vi "Wind_Tunnel.vi"() -> ()   [LabVIEW 2025]
uses:
  <vilib>/express/express arith-compare/Formula/XNode/ExpressFormulaBlockNode.xnode
panel:
  out "mph":dbl
  out "10":dbl(graph)
  out "Waveform Chart 2":dbl(graph)
  out "5":dbl(graph)
  out "m/s":dbl
  out "Numeric":dbl
  out "ma 10":dbl
  out "?":dbl
  out "PSIG 10":dbl(knob) scale=-2.0..5.0
  out "ma 9":dbl
  out "?":dbl
  out "PSIG 9":dbl(knob) scale=-2.0..5.0
  out "ma 8":dbl
  out "?":dbl
  out "PSIG 8":dbl(knob) scale=-2.0..5.0
  out "ma 7":dbl
  out "?":dbl
  out "PSIG 7":dbl(knob) scale=-2.0..5.0
  out "ma 6":dbl
  out "?":dbl
  out "PSIG 6":dbl(knob) scale=-2.0..5.0
  out "ma 5":dbl
  out "?":dbl
  out "PSIG 5":dbl(knob) scale=-2.0..5.0
  out "ma 4":dbl
  out "?":dbl
  out "PSIG 4":dbl(knob) scale=-2.0..5.0
  out "ma 3":dbl
  out "?":dbl
  out "PSIG 3":dbl(knob) scale=-2.0..5.0
  out "ma 2":dbl
  out "?":dbl
  out "PSIG 2":dbl(knob) scale=-2.0..5.0
  out "ma":dbl
  out "?":dbl
  out "PSIG":dbl(knob) scale=-2.0..5.0
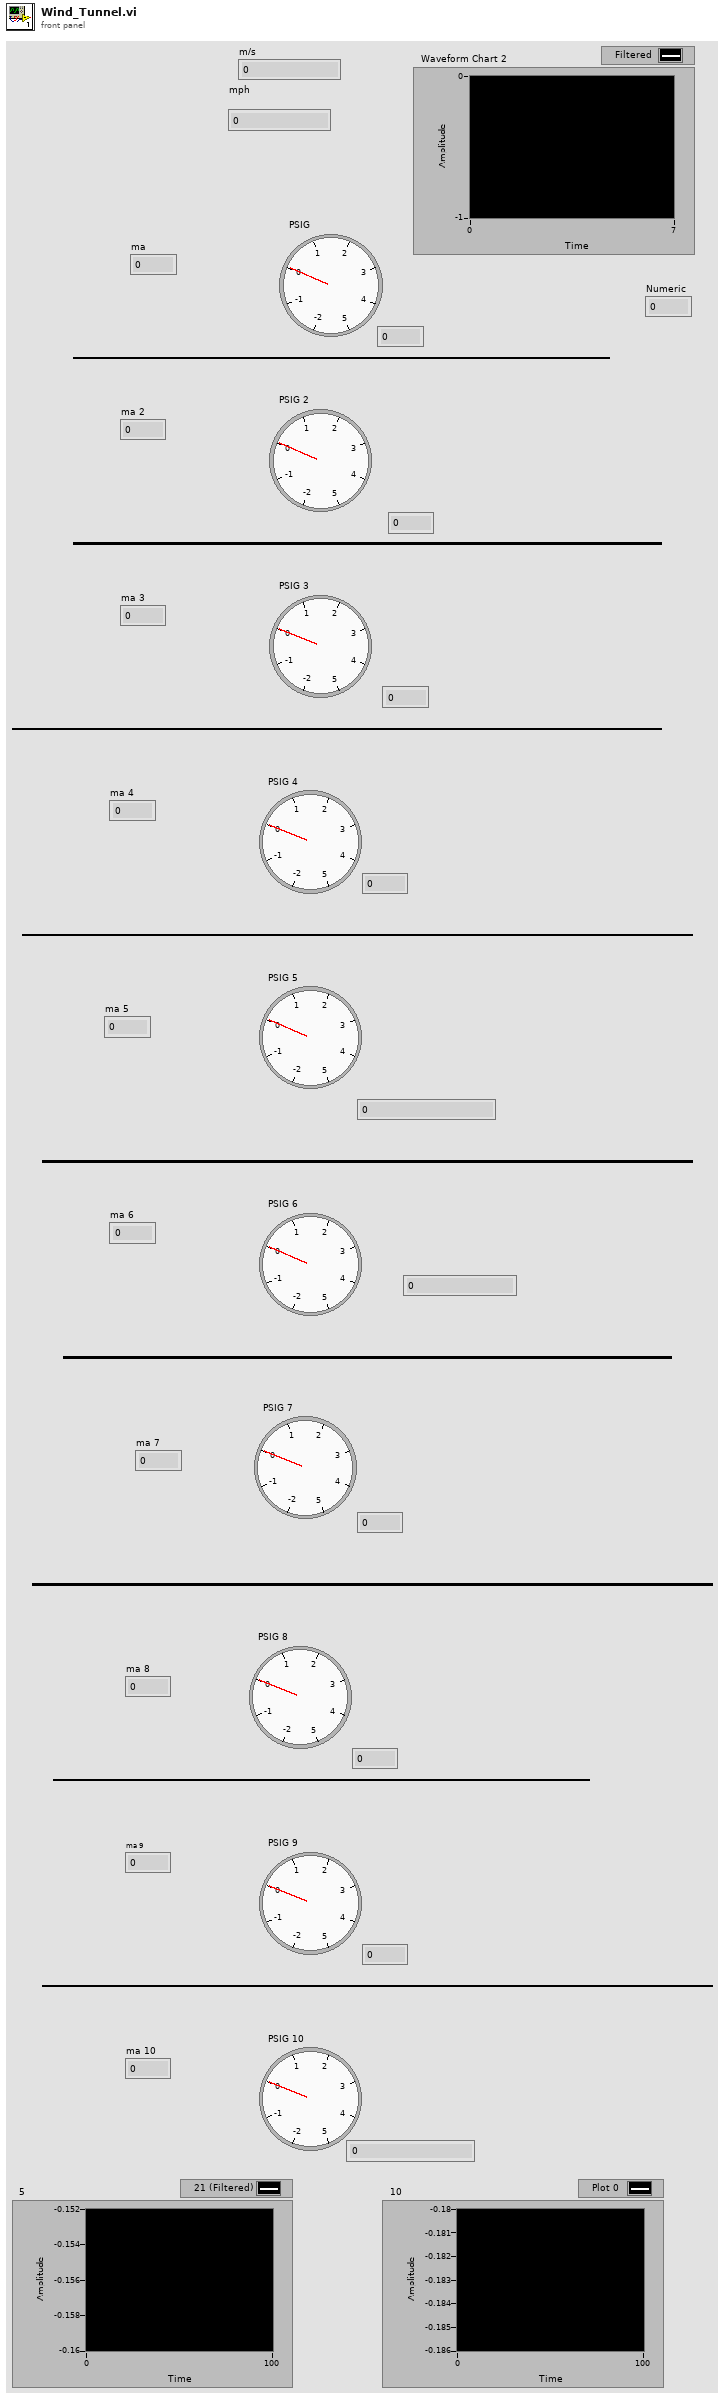
[diagram p1: front panel]
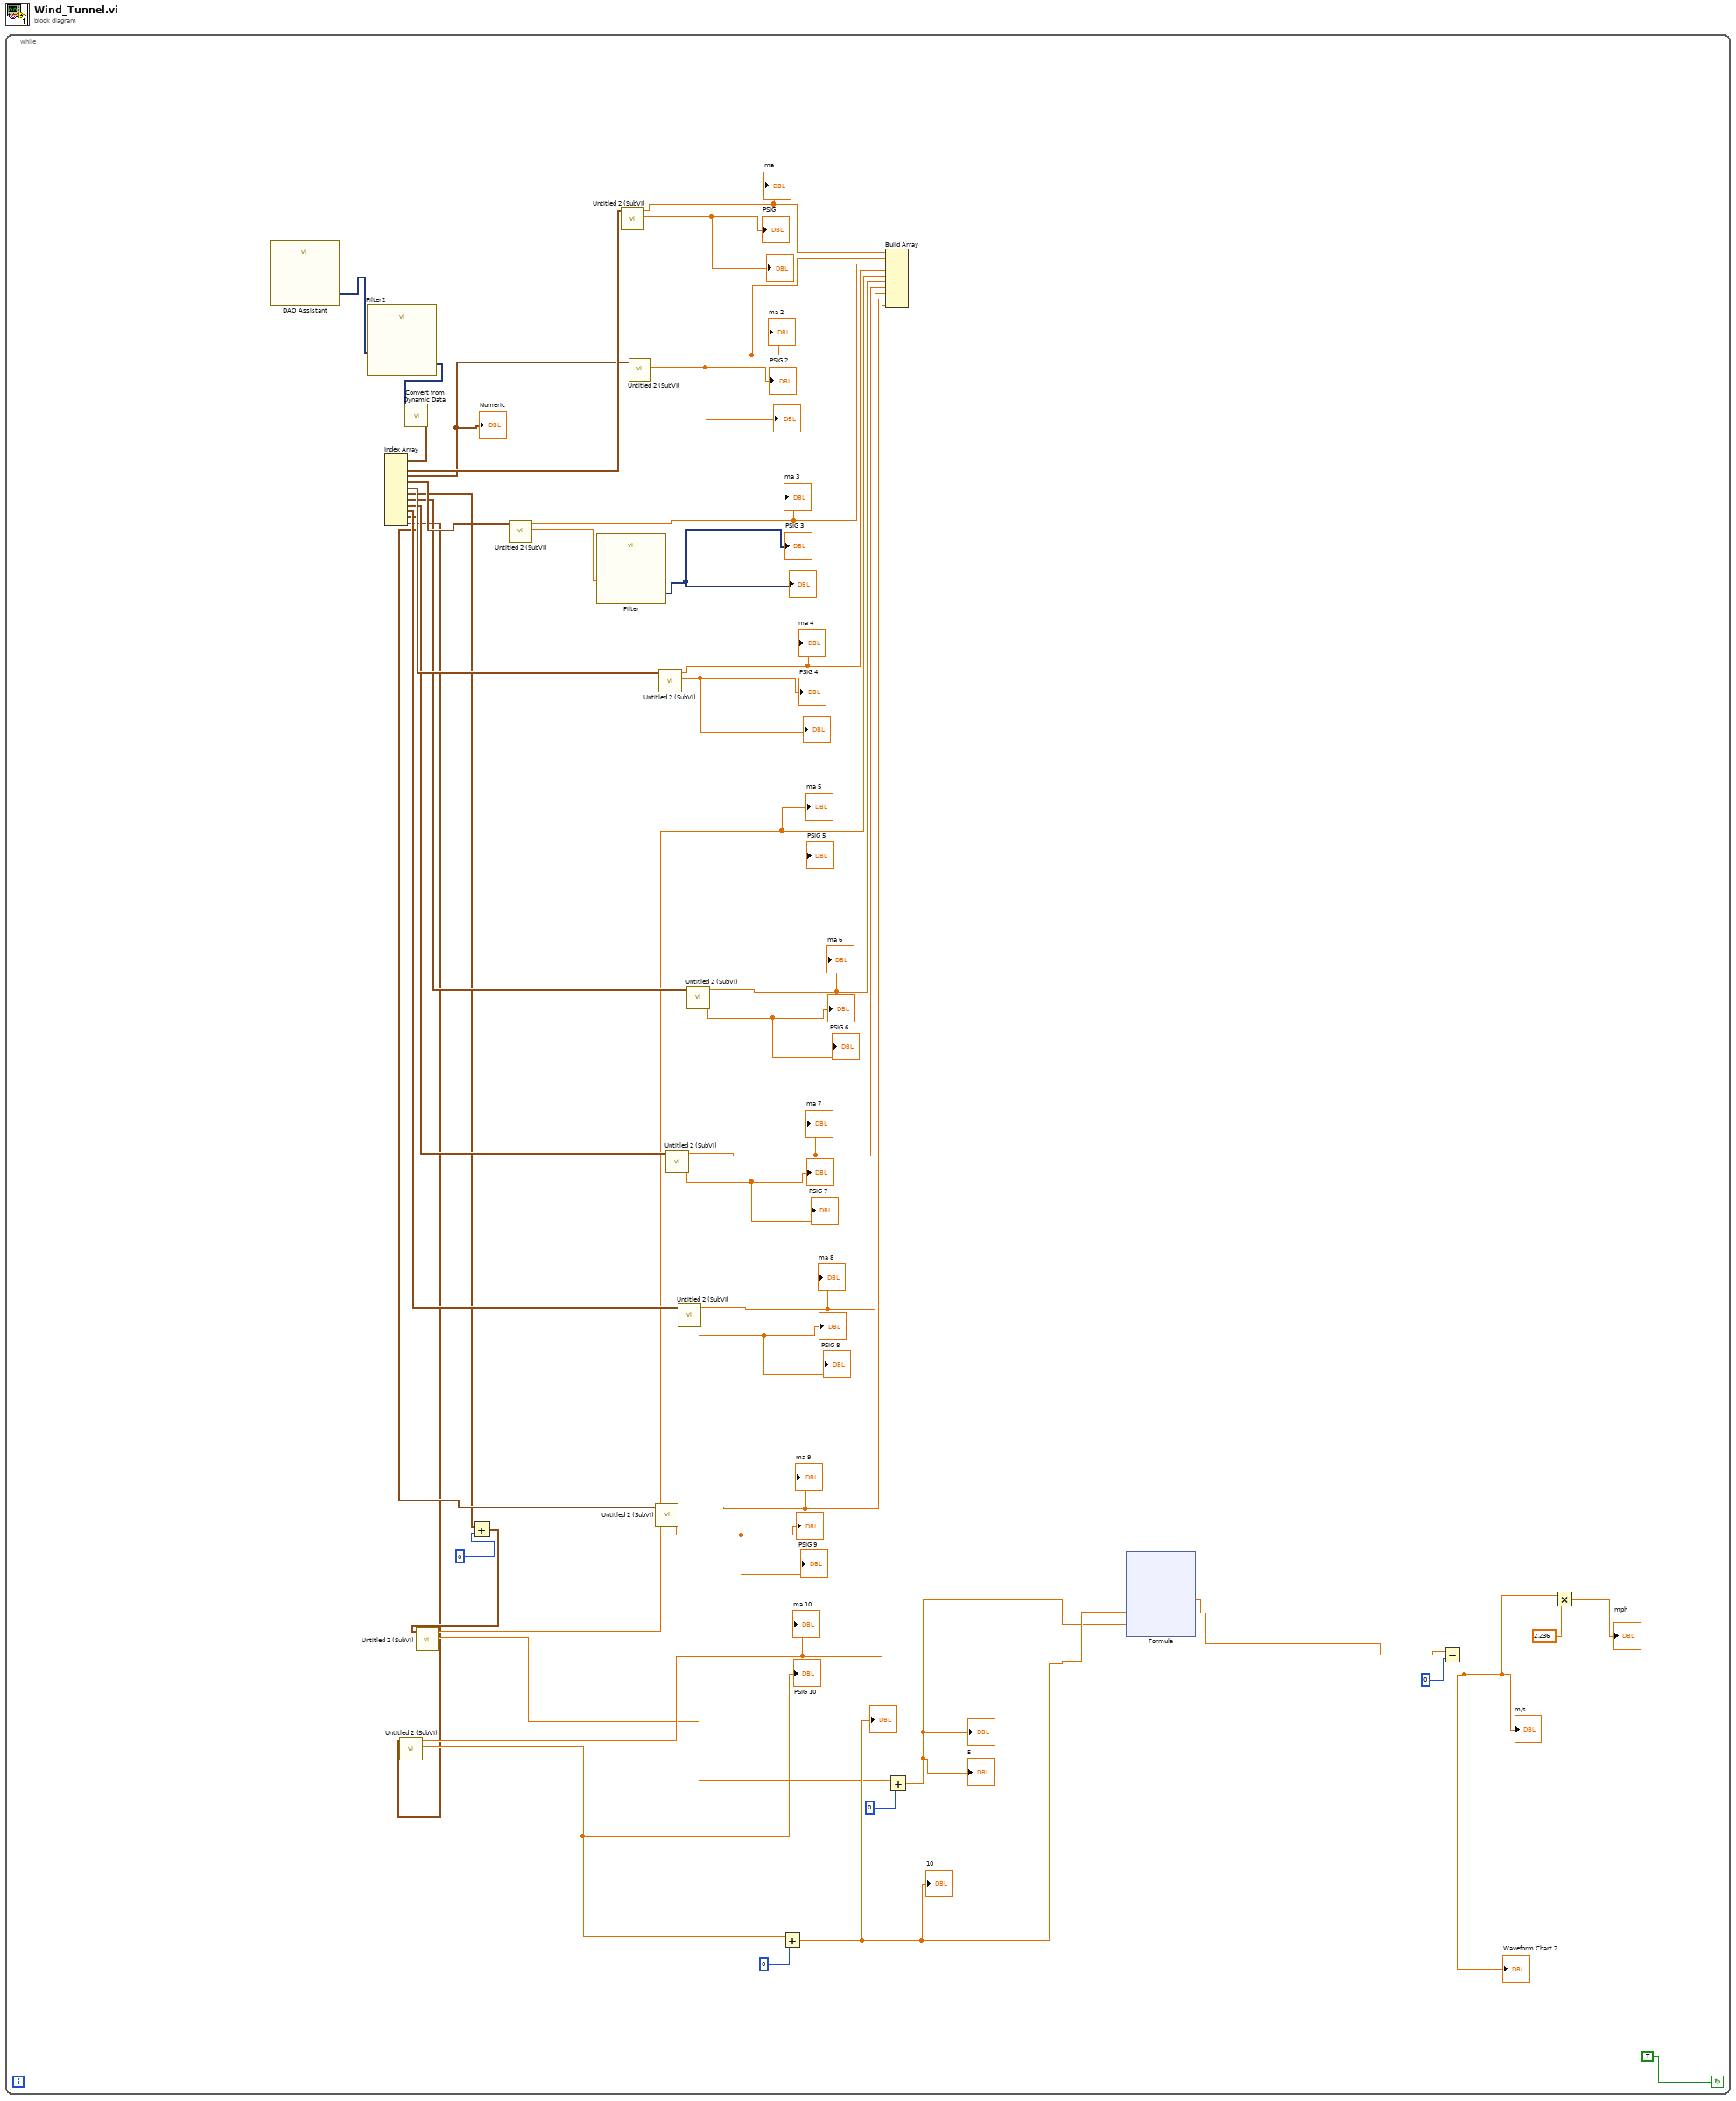
[diagram p0: block diagram]
diagram:
  n1 = while {
    stop <- TRUE continue-if-true
    n2 = call "DAQ Assistant"() -> ("data"=w1:dynamicdata)  [unwired: 16 in, 3 out]
    n3 = call "Filter2"("Signal"=w1) -> ("Filtered Signal"=w4:dynamicdata)  [unwired: 9 in, 1 out]
    n4 = call "Convert from Dynamic Data"("Dynamic Data Type"=w4) -> ("Array of Waveform"=w10:waveform(dbl)[])  [unwired: 3 in]
    n5 = Index Array(array=w10) -> (element #1=w46:waveform(dbl), element #2=w24:waveform(dbl), element #3=w40:waveform(dbl), element #4=w42:waveform(dbl), element #5=w9:waveform(dbl), element #6=w39:waveform(dbl), element #7=w36:waveform(dbl), element #8=w35:waveform(dbl), element #9=w33:waveform(dbl), element #10=w5:waveform(dbl))  [unwired: 10 in]
    "Numeric" <- w24
    n6 = call "Untitled 2 (SubVI).vi"("Numeric"=w5) -> ("PSIG"=w6:dbl, "ma"=w22:dbl)  [unwired: 8 in, 1 out]
    "PSIG 10" <- w6
    "ma 10" <- w22
    n7 = Add(x=w9, y=0) -> (x+y=w8:waveform(dbl))
    n8 = call "Untitled 2 (SubVI).vi"("Numeric"=w8) -> ("PSIG"=w7:dbl, "ma"=w21:dbl)  [unwired: 8 in, 1 out]
    "ma 5" <- w21
    n9 = call "Untitled 2 (SubVI).vi"("Numeric"=w40) -> ("PSIG"=w23:dbl, "ma"=w30:dbl)  [unwired: 8 in, 1 out]
    "ma 3" <- w30
    n10 = call "Filter"("Signal"=w23) -> ("Filtered Signal"=→"PSIG 3" →"?":dynamicdata)  [unwired: 9 in, 1 out]
    n11 = call "Untitled 2 (SubVI).vi"("Numeric"=w46) -> ("PSIG"=→"PSIG" →"?":dbl, "ma"=w32:dbl)  [unwired: 8 in, 1 out]
    "ma" <- w32
    n12 = call "Untitled 2 (SubVI).vi"("Numeric"=w24) -> ("PSIG"=→"PSIG 2" →"?":dbl, "ma"=w31:dbl)  [unwired: 8 in, 1 out]
    "ma 2" <- w31
    n13 = call "Untitled 2 (SubVI).vi"("Numeric"=w33) -> ("PSIG"=→"PSIG 9" →"?":dbl, "ma"=w25:dbl)  [unwired: 8 in, 1 out]
    "ma 9" <- w25
    n14 = call "Untitled 2 (SubVI).vi"("Numeric"=w42) -> ("PSIG"=→"PSIG 4" →"?":dbl, "ma"=w29:dbl)  [unwired: 8 in, 1 out]
    "ma 4" <- w29
    n15 = call "Untitled 2 (SubVI).vi"("Numeric"=w36) -> ("PSIG"=→"PSIG 7" →"?":dbl, "ma"=w27:dbl)  [unwired: 8 in, 1 out]
    "ma 7" <- w27
    n16 = call "Untitled 2 (SubVI).vi"("Numeric"=w35) -> ("PSIG"=→"PSIG 8" →"?":dbl, "ma"=w26:dbl)  [unwired: 8 in, 1 out]
    "ma 8" <- w26
    n17 = call "Untitled 2 (SubVI).vi"("Numeric"=w39) -> ("PSIG"=→"PSIG 6" →"?":dbl, "ma"=w28:dbl)  [unwired: 8 in, 1 out]
    "ma 6" <- w28
    n18 = Add(x=w6, y=0) -> (x+y=w15:dbl)
    "?" <- w15
    "10" <- w15
    n19 = Build Array(w32, w31, w30, w29, w21, w28, w27, w26, w25, w22) -> ()  [unwired: 1 out]
    n20 = Add(x=w7, y=0) -> (x+y=w14:dbl)
    "?" <- w14
    "5" <- w14
    n21 = xnode "Formula"("T"=w15, "S"=w14) -> ("Result"=w3:dbl)  [unwired: 1 in, 1 out]
    n22 = Subtract(x=w3, y=0) -> (x-y=w12:dbl)
    "m/s" <- w12
    "Waveform Chart 2" <- w12
    n23 = Multiply(x=w12, y=2.236) -> (x*y=→"mph":dbl)
  }
